vi "S4GUI_001.vi"() -> ()   [LabVIEW 2018] (continued)
                n1814 = call-dynamic "Get CCD_Config.vi"("error in (no error)"=w4172, "Interface in"=w4173) -> ("error out"=w4221:errorcluster, "output cluster"=w4222:T24, "Interface out"=w4218:refnum<class "Interface.lvclass">)  [unwired: 7 in]
                n1815 = Bundle By Name(cluster=w4222, "SHUTTER_MODE"=u8 2, "FRAME_TRANSFER"=w4171) -> (w4220:T24)
                n1816 = call-dynamic "Set CCD_Config.vi"("error in (no error)"=w4221, "input cluster"=w4220, "Interface in"=w4218) -> ("error out"=w4223:errorcluster, "Interface out"=w4217:refnum<class "Interface.lvclass">)  [unwired: 7 in]
                n1817 = Flatten To String(anything=w4220, error in (no error)=w4223) -> (data string=w4225:string, error out=w4224:errorcluster)  [unwired: 2 in, 1 out]
                n1818 = call "Write flatted cluster.vi"("error in (no error)"=w4224, "flatted cluster"=w4225, "Interface in"=w4217) -> ("error out"=w4215:errorcluster, "Interface out"=w4216:refnum<class "Interface.lvclass">)  [unwired: 7 in]
                n1819 = call-dynamic "Write Interface.vi"("error in (no error)"=w4215, "Interface.lvclass"=w4216, "Channel in"=w4229) -> ("error out"=w4210:errorcluster, "Channel out"=w4209:refnum<class "Channel.lvclass">)  [unwired: 7 in]
                n1820 = call "Write section_name.vi"("error in (no error)"=w4210, "section_name"="CCD_ACS4", "Channel in"=w4209) -> ("error out"=w4211:errorcluster, "Channel out"=w4206:refnum<class "Channel.lvclass">)  [unwired: 7 in]
                n1821 = call-dynamic "save config.vi"("error in (no error)"=w4211, "file config"="lastsaved.cfg", "Channel in"=w4206) -> ("error out"=w4179:errorcluster, "Channel out"=w4180:refnum<class "Channel.lvclass">)  [unwired: 7 in]
                n1822 = local read "Filter4"() -> (w4181:u8)
                n1823 = call-dynamic "Write Filter.vi"("error in (no error)"=w4179, "Filter"=w4181, "Channel in"=w4180) -> ("error out"=w4188:errorcluster, "Channel out"=w4189:refnum<class "Channel.lvclass">)  [unwired: 7 in]
                n1824 = call-dynamic "Read Interface.vi"("error in (no error)"=w4188, "Channel in"=w4189) -> ("error out"=w4186:errorcluster, "Interface.lvclass"=w4191:refnum<class "Interface.lvclass">, "Channel out"=w4190:refnum<class "Channel.lvclass">)  [unwired: 7 in]
                n1825 = call-dynamic "Write Suffix.vi"("error in (no error)"=w4186, "Suffix"=w4168, "Interface in"=w4191) -> ("error out"=w4182:errorcluster, "Interface out"=w4192:refnum<class "Interface.lvclass">)  [unwired: 7 in]
                n1826 = call-dynamic "Write ObsType.vi"("error in (no error)"=w4182, "ObsType"=w4167, "Interface in"=w4192) -> ("error out"=w4183:errorcluster, "Interface out"=w4193:refnum<class "Interface.lvclass">)  [unwired: 7 in]
                n1827 = call-dynamic "Write Object.vi"("error in (no error)"=w4183, "Object"=w4176, "Interface in"=w4193) -> ("error out"=w4184:errorcluster, "Interface out"=w4194:refnum<class "Interface.lvclass">)  [unwired: 7 in]
                n1828 = call-dynamic "Write Comments.vi"("error in (no error)"=w4184, "Comments"=w4175, "Interface in"=w4194) -> ("error out"=w4185:errorcluster, "Interface out"=w4195:refnum<class "Interface.lvclass">)  [unwired: 7 in]
                n1829 = call-dynamic "Write Observer.vi"("error in (no error)"=w4185, "Observer"=w4174, "Interface in"=w4195) -> ("error out"=w4187:errorcluster, "Interface out"=w4196:refnum<class "Interface.lvclass">)  [unwired: 7 in]
                n1830 = call-dynamic "Write Interface.vi"("error in (no error)"=w4187, "Interface.lvclass"=w4196, "Channel in"=w4190) -> ("error out"=w4177:errorcluster, "Channel out"=w4178:refnum<class "Channel.lvclass">)  [unwired: 7 in]
                n1831 = call-dynamic "Read State Machine.vi"("error in (no error)"=w4177, "Device in"=w4178) -> ("error out"=w4214:errorcluster, "State Machine.lvclass"=w4204:refnum<class "State Machine.lvclass">, "Device out"=w4205:refnum<class "Channel.lvclass">)  [unwired: 7 in]
                n1832 = call-dynamic "Write State.vi"("error in (no error)"=w4214, "State"=60, "State Machine in"=w4204) -> ("error out"=w4213:errorcluster, "State Machine out"=w4203:refnum<class "State Machine.lvclass">)  [unwired: 7 in]
                n1833 = call-dynamic "Write State Machine.vi"("error in (no error)"=w4213, "State Machine.lvclass"=w4203, "Device in"=w4205) -> ("error out"=w4202:errorcluster, "Device out"=w4197:refnum<class "Channel.lvclass">)  [unwired: 7 in]
                n1834 = call-dynamic "Write Channel.vi"("error in (no error)"=w4202, "Channel.lvclass"=w4197, "Acquisition in"=w4228) -> ("error out"=w4198:errorcluster, "Acquisition out"=w4199:refnum<class "Acquisition.lvclass">)  [unwired: 7 in]
              }
            }
            n1835 = case shown="True" w4144 {
              tunnel: w4146 -> [w4321 w4360]
              tunnel: w4145 -> [w4320 w4359]
              tunnel: [w4321 w4358] -> w4157
              tunnel: [w4320 w4357] -> w4156
              tunnel: w4131 -> [_ w4336]
              tunnel: w4130 -> [_ w4335]
              tunnel: w4129 -> [_ w4334]
              tunnel: w4128 -> [_ w4328]
              tunnel: w4127 -> [_ w4327]
              frame False {
              }
              frame True {
                # "nome do arquivo .cfg"
                # "seção no arquivo .cfg"
                # "closed"
                n1836 = call-dynamic "Read Channel.vi"("error in (no error)"=w4359, "Acquisition in"=w4360) -> ("error out"=w4364:errorcluster, "Channel.lvclass"=w4363:refnum<class "Channel.lvclass">, "Acquisition out"=w4362:refnum<class "Acquisition.lvclass">)  [unwired: 7 in]
                n1837 = call-dynamic "Read Interface.vi"("error in (no error)"=w4364, "Channel in"=w4363) -> ("error out"=w4326:errorcluster, "Interface.lvclass"=w4325:refnum<class "Interface.lvclass">, "Channel out"=w4361:refnum<class "Channel.lvclass">)  [unwired: 7 in]
                n1838 = call-dynamic "Read restoreExpTime.vi"("error in (no error)"=w4326, "Interface in"=w4325) -> ("error out"=w4323:errorcluster, "restoreExpTime"=w4322:bool, "Interface out"=w4324:refnum<class "Interface.lvclass">)  [unwired: 7 in]
                n1839 = case shown="True" w4322 {
                  tunnel: w4324 -> [w4391 w4396]
                  tunnel: [w4391 w4399] -> w4330
                  tunnel: w4323 -> [w4390 w4394]
                  tunnel: [w4390 w4398] -> w4329
                  frame False {
                  }
                  frame True {
                    n1840 = call-dynamic "Write restoreExpTime.vi"("error in (no error)"=w4394, "restoreExpTime"=FALSE, "Interface in"=w4396) -> ("error out"=w4393:errorcluster, "Interface out"=w4395:refnum<class "Interface.lvclass">)  [unwired: 7 in]
                    n1841 = call-dynamic "Read prev ExpTime.vi"("error in (no error)"=w4393, "Interface in"=w4395) -> ("error out"=w4398:errorcluster, "prev ExpTime"=w4397:dbl, "Interface out"=w4399:refnum<class "Interface.lvclass">)  [unwired: 7 in]
                    n1842 = property on="Exptime ch2" class="DigNum (strict)"("Value"=w4397) -> ()  [unwired: 2 in, 2 out]
                  }
                }
                n1843 = call-dynamic "Read PREV_FT.vi"("error in (no error)"=w4329, "Interface in"=w4330) -> ("error out"=w4332:errorcluster, "PREV_FT"=w4331:bool, "Interface out"=w4333:refnum<class "Interface.lvclass">)  [unwired: 7 in]
                n1844 = call-dynamic "Get CCD_Config.vi"("error in (no error)"=w4332, "Interface in"=w4333) -> ("error out"=w4369:errorcluster, "output cluster"=w4368:T24, "Interface out"=w4372:refnum<class "Interface.lvclass">)  [unwired: 7 in]
                n1845 = Bundle By Name(cluster=w4368, "SHUTTER_MODE"=u8 2, "FRAME_TRANSFER"=w4331) -> (w4370:T24)
                n1846 = call-dynamic "Set CCD_Config.vi"("error in (no error)"=w4369, "input cluster"=w4370, "Interface in"=w4372) -> ("error out"=w4367:errorcluster, "Interface out"=w4373:refnum<class "Interface.lvclass">)  [unwired: 7 in]
                n1847 = Flatten To String(anything=w4370, error in (no error)=w4367) -> (data string=w4365:string, error out=w4366:errorcluster)  [unwired: 2 in, 1 out]
                n1848 = call "Write flatted cluster.vi"("error in (no error)"=w4366, "flatted cluster"=w4365, "Interface in"=w4373) -> ("error out"=w4375:errorcluster, "Interface out"=w4374:refnum<class "Interface.lvclass">)  [unwired: 7 in]
                n1849 = call-dynamic "Write Interface.vi"("error in (no error)"=w4375, "Interface.lvclass"=w4374, "Channel in"=w4361) -> ("error out"=w4380:errorcluster, "Channel out"=w4381:refnum<class "Channel.lvclass">)  [unwired: 7 in]
                n1850 = call "Write section_name.vi"("error in (no error)"=w4380, "section_name"="CCD_ACS2", "Channel in"=w4381) -> ("error out"=w4379:errorcluster, "Channel out"=w4384:refnum<class "Channel.lvclass">)  [unwired: 7 in]
                n1851 = call-dynamic "save config.vi"("error in (no error)"=w4379, "file config"="lastsaved.cfg", "Channel in"=w4384) -> ("error out"=w4339:errorcluster, "Channel out"=w4340:refnum<class "Channel.lvclass">)  [unwired: 7 in]
                n1852 = local read "Filter2"() -> (w4341:u8)
                n1853 = call-dynamic "Write Filter.vi"("error in (no error)"=w4339, "Filter"=w4341, "Channel in"=w4340) -> ("error out"=w4348:errorcluster, "Channel out"=w4349:refnum<class "Channel.lvclass">)  [unwired: 7 in]
                n1854 = call-dynamic "Read Interface.vi"("error in (no error)"=w4348, "Channel in"=w4349) -> ("error out"=w4346:errorcluster, "Interface.lvclass"=w4351:refnum<class "Interface.lvclass">, "Channel out"=w4350:refnum<class "Channel.lvclass">)  [unwired: 7 in]
                n1855 = call-dynamic "Write Suffix.vi"("error in (no error)"=w4346, "Suffix"=w4328, "Interface in"=w4351) -> ("error out"=w4342:errorcluster, "Interface out"=w4352:refnum<class "Interface.lvclass">)  [unwired: 7 in]
                n1856 = call-dynamic "Write ObsType.vi"("error in (no error)"=w4342, "ObsType"=w4327, "Interface in"=w4352) -> ("error out"=w4343:errorcluster, "Interface out"=w4353:refnum<class "Interface.lvclass">)  [unwired: 7 in]
                n1857 = call-dynamic "Write Object.vi"("error in (no error)"=w4343, "Object"=w4336, "Interface in"=w4353) -> ("error out"=w4344:errorcluster, "Interface out"=w4354:refnum<class "Interface.lvclass">)  [unwired: 7 in]
                n1858 = call-dynamic "Write Comments.vi"("error in (no error)"=w4344, "Comments"=w4335, "Interface in"=w4354) -> ("error out"=w4345:errorcluster, "Interface out"=w4355:refnum<class "Interface.lvclass">)  [unwired: 7 in]
                n1859 = call-dynamic "Write Observer.vi"("error in (no error)"=w4345, "Observer"=w4334, "Interface in"=w4355) -> ("error out"=w4347:errorcluster, "Interface out"=w4356:refnum<class "Interface.lvclass">)  [unwired: 7 in]
                n1860 = call-dynamic "Write Interface.vi"("error in (no error)"=w4347, "Interface.lvclass"=w4356, "Channel in"=w4350) -> ("error out"=w4337:errorcluster, "Channel out"=w4338:refnum<class "Channel.lvclass">)  [unwired: 7 in]
                n1861 = call-dynamic "Read State Machine.vi"("error in (no error)"=w4337, "Device in"=w4338) -> ("error out"=w4376:errorcluster, "State Machine.lvclass"=w4386:refnum<class "State Machine.lvclass">, "Device out"=w4385:refnum<class "Channel.lvclass">)  [unwired: 7 in]
                n1862 = call-dynamic "Write State.vi"("error in (no error)"=w4376, "State"=60, "State Machine in"=w4386) -> ("error out"=w4377:errorcluster, "State Machine out"=w4387:refnum<class "State Machine.lvclass">)  [unwired: 7 in]
                n1863 = call-dynamic "Write State Machine.vi"("error in (no error)"=w4377, "State Machine.lvclass"=w4387, "Device in"=w4385) -> ("error out"=w4389:errorcluster, "Device out"=w4388:refnum<class "Channel.lvclass">)  [unwired: 7 in]
                n1864 = call-dynamic "Write Channel.vi"("error in (no error)"=w4389, "Channel.lvclass"=w4388, "Acquisition in"=w4362) -> ("error out"=w4357:errorcluster, "Acquisition out"=w4358:refnum<class "Acquisition.lvclass">)  [unwired: 7 in]
              }
            }
            n1865 = case shown="True" w4141 {
              tunnel: w4143 -> [w4241 w4280]
              tunnel: w4142 -> [w4240 w4279]
              tunnel: [w4241 w4278] -> w4155
              tunnel: [w4240 w4277] -> w4154
              tunnel: w4131 -> [_ w4256]
              tunnel: w4130 -> [_ w4255]
              tunnel: w4129 -> [_ w4254]
              tunnel: w4128 -> [_ w4248]
              tunnel: w4127 -> [_ w4247]
              frame False {
              }
              frame True {
                # "nome do arquivo .cfg"
                # "seção no arquivo .cfg"
                # "closed"
                n1866 = call-dynamic "Read Channel.vi"("error in (no error)"=w4279, "Acquisition in"=w4280) -> ("error out"=w4284:errorcluster, "Channel.lvclass"=w4283:refnum<class "Channel.lvclass">, "Acquisition out"=w4282:refnum<class "Acquisition.lvclass">)  [unwired: 7 in]
                n1867 = call-dynamic "Read Interface.vi"("error in (no error)"=w4284, "Channel in"=w4283) -> ("error out"=w4244:errorcluster, "Interface.lvclass"=w4246:refnum<class "Interface.lvclass">, "Channel out"=w4281:refnum<class "Channel.lvclass">)  [unwired: 7 in]
                n1868 = call-dynamic "Read restoreExpTime.vi"("error in (no error)"=w4244, "Interface in"=w4246) -> ("error out"=w4243:errorcluster, "restoreExpTime"=w4242:bool, "Interface out"=w4245:refnum<class "Interface.lvclass">)  [unwired: 7 in]
                n1869 = case shown="True" w4242 {
                  tunnel: w4245 -> [w4311 w4316]
                  tunnel: [w4311 w4319] -> w4250
                  tunnel: w4243 -> [w4310 w4315]
                  tunnel: [w4310 w4318] -> w4249
                  frame False {
                  }
                  frame True {
                    n1870 = call-dynamic "Write restoreExpTime.vi"("error in (no error)"=w4315, "restoreExpTime"=FALSE, "Interface in"=w4316) -> ("error out"=w4312:errorcluster, "Interface out"=w4313:refnum<class "Interface.lvclass">)  [unwired: 7 in]
                    n1871 = call-dynamic "Read prev ExpTime.vi"("error in (no error)"=w4312, "Interface in"=w4313) -> ("error out"=w4318:errorcluster, "prev ExpTime"=w4317:dbl, "Interface out"=w4319:refnum<class "Interface.lvclass">)  [unwired: 7 in]
                    n1872 = property on="Exptime ch3" class="DigNum (strict)"("Value"=w4317) -> ()  [unwired: 2 in, 2 out]
                  }
                }
                n1873 = call-dynamic "Read PREV_FT.vi"("error in (no error)"=w4249, "Interface in"=w4250) -> ("error out"=w4252:errorcluster, "PREV_FT"=w4251:bool, "Interface out"=w4253:refnum<class "Interface.lvclass">)  [unwired: 7 in]
                n1874 = call-dynamic "Get CCD_Config.vi"("error in (no error)"=w4252, "Interface in"=w4253) -> ("error out"=w4289:errorcluster, "output cluster"=w4288:T24, "Interface out"=w4292:refnum<class "Interface.lvclass">)  [unwired: 7 in]
                n1875 = Bundle By Name(cluster=w4288, "SHUTTER_MODE"=u8 2, "FRAME_TRANSFER"=w4251) -> (w4290:T24)
                n1876 = call-dynamic "Set CCD_Config.vi"("error in (no error)"=w4289, "input cluster"=w4290, "Interface in"=w4292) -> ("error out"=w4287:errorcluster, "Interface out"=w4293:refnum<class "Interface.lvclass">)  [unwired: 7 in]
                n1877 = Flatten To String(anything=w4290, error in (no error)=w4287) -> (data string=w4285:string, error out=w4286:errorcluster)  [unwired: 2 in, 1 out]
                n1878 = call "Write flatted cluster.vi"("error in (no error)"=w4286, "flatted cluster"=w4285, "Interface in"=w4293) -> ("error out"=w4295:errorcluster, "Interface out"=w4294:refnum<class "Interface.lvclass">)  [unwired: 7 in]
                n1879 = call-dynamic "Write Interface.vi"("error in (no error)"=w4295, "Interface.lvclass"=w4294, "Channel in"=w4281) -> ("error out"=w4300:errorcluster, "Channel out"=w4301:refnum<class "Channel.lvclass">)  [unwired: 7 in]
                n1880 = call "Write section_name.vi"("error in (no error)"=w4300, "section_name"="CCD_ACS3", "Channel in"=w4301) -> ("error out"=w4299:errorcluster, "Channel out"=w4304:refnum<class "Channel.lvclass">)  [unwired: 7 in]
                n1881 = call-dynamic "save config.vi"("error in (no error)"=w4299, "file config"="lastsaved.cfg", "Channel in"=w4304) -> ("error out"=w4259:errorcluster, "Channel out"=w4260:refnum<class "Channel.lvclass">)  [unwired: 7 in]
                n1882 = local read "Filter3"() -> (w4261:u8)
                n1883 = call-dynamic "Write Filter.vi"("error in (no error)"=w4259, "Filter"=w4261, "Channel in"=w4260) -> ("error out"=w4268:errorcluster, "Channel out"=w4269:refnum<class "Channel.lvclass">)  [unwired: 7 in]
                n1884 = call-dynamic "Read Interface.vi"("error in (no error)"=w4268, "Channel in"=w4269) -> ("error out"=w4266:errorcluster, "Interface.lvclass"=w4271:refnum<class "Interface.lvclass">, "Channel out"=w4270:refnum<class "Channel.lvclass">)  [unwired: 7 in]
                n1885 = call-dynamic "Write Suffix.vi"("error in (no error)"=w4266, "Suffix"=w4248, "Interface in"=w4271) -> ("error out"=w4262:errorcluster, "Interface out"=w4272:refnum<class "Interface.lvclass">)  [unwired: 7 in]
                n1886 = call-dynamic "Write ObsType.vi"("error in (no error)"=w4262, "ObsType"=w4247, "Interface in"=w4272) -> ("error out"=w4263:errorcluster, "Interface out"=w4273:refnum<class "Interface.lvclass">)  [unwired: 7 in]
                n1887 = call-dynamic "Write Object.vi"("error in (no error)"=w4263, "Object"=w4256, "Interface in"=w4273) -> ("error out"=w4264:errorcluster, "Interface out"=w4274:refnum<class "Interface.lvclass">)  [unwired: 7 in]
                n1888 = call-dynamic "Write Comments.vi"("error in (no error)"=w4264, "Comments"=w4255, "Interface in"=w4274) -> ("error out"=w4265:errorcluster, "Interface out"=w4275:refnum<class "Interface.lvclass">)  [unwired: 7 in]
                n1889 = call-dynamic "Write Observer.vi"("error in (no error)"=w4265, "Observer"=w4254, "Interface in"=w4275) -> ("error out"=w4267:errorcluster, "Interface out"=w4276:refnum<class "Interface.lvclass">)  [unwired: 7 in]
                n1890 = call-dynamic "Write Interface.vi"("error in (no error)"=w4267, "Interface.lvclass"=w4276, "Channel in"=w4270) -> ("error out"=w4257:errorcluster, "Channel out"=w4258:refnum<class "Channel.lvclass">)  [unwired: 7 in]
                n1891 = call-dynamic "Read State Machine.vi"("error in (no error)"=w4257, "Device in"=w4258) -> ("error out"=w4296:errorcluster, "State Machine.lvclass"=w4306:refnum<class "State Machine.lvclass">, "Device out"=w4305:refnum<class "Channel.lvclass">)  [unwired: 7 in]
                n1892 = call-dynamic "Write State.vi"("error in (no error)"=w4296, "State"=60, "State Machine in"=w4306) -> ("error out"=w4297:errorcluster, "State Machine out"=w4307:refnum<class "State Machine.lvclass">)  [unwired: 7 in]
                n1893 = call-dynamic "Write State Machine.vi"("error in (no error)"=w4297, "State Machine.lvclass"=w4307, "Device in"=w4305) -> ("error out"=w4309:errorcluster, "Device out"=w4308:refnum<class "Channel.lvclass">)  [unwired: 7 in]
                n1894 = call-dynamic "Write Channel.vi"("error in (no error)"=w4309, "Channel.lvclass"=w4308, "Acquisition in"=w4282) -> ("error out"=w4277:errorcluster, "Acquisition out"=w4278:refnum<class "Acquisition.lvclass">)  [unwired: 7 in]
              }
            }
            n1895 = case shown="True" w4147 {
              tunnel: [w4400 w4465] -> w4158
              tunnel: [w4401 w4464] -> w4159
              tunnel: w4149 -> [w4401 w4438]
              tunnel: w4148 -> [w4400 w4437]
              tunnel: w4131 -> [_ w4416]
              tunnel: w4130 -> [_ w4415]
              tunnel: w4129 -> [_ w4414]
              tunnel: w4128 -> [_ w4408]
              tunnel: w4127 -> [_ w4407]
              frame False {
              }
              frame True {
                # "nome do arquivo .cfg"
                # "seção no arquivo .cfg"
                # "closed"
                n1896 = call-dynamic "Read Channel.vi"("error in (no error)"=w4437, "Acquisition in"=w4438) -> ("error out"=w4466:errorcluster, "Channel.lvclass"=w4467:refnum<class "Channel.lvclass">, "Acquisition out"=w4468:refnum<class "Acquisition.lvclass">)  [unwired: 7 in]
                n1897 = call-dynamic "Read Interface.vi"("error in (no error)"=w4466, "Channel in"=w4467) -> ("error out"=w4405:errorcluster, "Interface.lvclass"=w4406:refnum<class "Interface.lvclass">, "Channel out"=w4469:refnum<class "Channel.lvclass">)  [unwired: 7 in]
                n1898 = call-dynamic "Read restoreExpTime.vi"("error in (no error)"=w4405, "Interface in"=w4406) -> ("error out"=w4403:errorcluster, "restoreExpTime"=w4402:bool, "Interface out"=w4404:refnum<class "Interface.lvclass">)  [unwired: 7 in]
                n1899 = case shown="True" w4402 {
                  tunnel: [w4471 w4479] -> w4410
                  tunnel: [w4470 w4478] -> w4409
                  tunnel: w4404 -> [w4471 w4476]
                  tunnel: w4403 -> [w4470 w4474]
                  frame False {
                  }
                  frame True {
                    n1900 = call-dynamic "Write restoreExpTime.vi"("error in (no error)"=w4474, "restoreExpTime"=FALSE, "Interface in"=w4476) -> ("error out"=w4473:errorcluster, "Interface out"=w4475:refnum<class "Interface.lvclass">)  [unwired: 7 in]
                    n1901 = call-dynamic "Read prev ExpTime.vi"("error in (no error)"=w4473, "Interface in"=w4475) -> ("error out"=w4478:errorcluster, "prev ExpTime"=w4477:dbl, "Interface out"=w4479:refnum<class "Interface.lvclass">)  [unwired: 7 in]
                    n1902 = property on="Exptime ch1" class="DigNum (strict)"("Value"=w4477) -> ()  [unwired: 2 in, 2 out]
                  }
                }
                n1903 = call-dynamic "Read PREV_FT.vi"("error in (no error)"=w4409, "Interface in"=w4410) -> ("error out"=w4412:errorcluster, "PREV_FT"=w4411:bool, "Interface out"=w4413:refnum<class "Interface.lvclass">)  [unwired: 7 in]
                n1904 = call-dynamic "Get CCD_Config.vi"("error in (no error)"=w4412, "Interface in"=w4413) -> ("error out"=w4459:errorcluster, "output cluster"=w4460:T24, "Interface out"=w4456:refnum<class "Interface.lvclass">)  [unwired: 7 in]
                n1905 = Bundle By Name(cluster=w4460, "SHUTTER_MODE"=u8 2, "FRAME_TRANSFER"=w4411) -> (w4458:T24)
                n1906 = call-dynamic "Set CCD_Config.vi"("error in (no error)"=w4459, "input cluster"=w4458, "Interface in"=w4456) -> ("error out"=w4461:errorcluster, "Interface out"=w4455:refnum<class "Interface.lvclass">)  [unwired: 7 in]
                n1907 = Flatten To String(anything=w4458, error in (no error)=w4461) -> (data string=w4463:string, error out=w4462:errorcluster)  [unwired: 2 in, 1 out]
                n1908 = call "Write flatted cluster.vi"("error in (no error)"=w4462, "flatted cluster"=w4463, "Interface in"=w4455) -> ("error out"=w4453:errorcluster, "Interface out"=w4454:refnum<class "Interface.lvclass">)  [unwired: 7 in]
                n1909 = call-dynamic "Write Interface.vi"("error in (no error)"=w4453, "Interface.lvclass"=w4454, "Channel in"=w4469) -> ("error out"=w4448:errorcluster, "Channel out"=w4447:refnum<class "Channel.lvclass">)  [unwired: 7 in]
                n1910 = call "Write section_name.vi"("error in (no error)"=w4448, "section_name"="CCD_ACS1", "Channel in"=w4447) -> ("error out"=w4449:errorcluster, "Channel out"=w4444:refnum<class "Channel.lvclass">)  [unwired: 7 in]
                n1911 = call-dynamic "save config.vi"("error in (no error)"=w4449, "file config"="lastsaved.cfg", "Channel in"=w4444) -> ("error out"=w4419:errorcluster, "Channel out"=w4420:refnum<class "Channel.lvclass">)  [unwired: 7 in]
                n1912 = local read "Filter1"() -> (w4421:u8)
                n1913 = call-dynamic "Write Filter.vi"("error in (no error)"=w4419, "Filter"=w4421, "Channel in"=w4420) -> ("error out"=w4428:errorcluster, "Channel out"=w4429:refnum<class "Channel.lvclass">)  [unwired: 7 in]
                n1914 = call-dynamic "Read Interface.vi"("error in (no error)"=w4428, "Channel in"=w4429) -> ("error out"=w4426:errorcluster, "Interface.lvclass"=w4431:refnum<class "Interface.lvclass">, "Channel out"=w4430:refnum<class "Channel.lvclass">)  [unwired: 7 in]
                n1915 = call-dynamic "Write Suffix.vi"("error in (no error)"=w4426, "Suffix"=w4408, "Interface in"=w4431) -> ("error out"=w4422:errorcluster, "Interface out"=w4432:refnum<class "Interface.lvclass">)  [unwired: 7 in]
                n1916 = call-dynamic "Write ObsType.vi"("error in (no error)"=w4422, "ObsType"=w4407, "Interface in"=w4432) -> ("error out"=w4423:errorcluster, "Interface out"=w4433:refnum<class "Interface.lvclass">)  [unwired: 7 in]
                n1917 = call-dynamic "Write Object.vi"("error in (no error)"=w4423, "Object"=w4416, "Interface in"=w4433) -> ("error out"=w4424:errorcluster, "Interface out"=w4434:refnum<class "Interface.lvclass">)  [unwired: 7 in]
                n1918 = call-dynamic "Write Comments.vi"("error in (no error)"=w4424, "Comments"=w4415, "Interface in"=w4434) -> ("error out"=w4425:errorcluster, "Interface out"=w4435:refnum<class "Interface.lvclass">)  [unwired: 7 in]
                n1919 = call-dynamic "Write Observer.vi"("error in (no error)"=w4425, "Observer"=w4414, "Interface in"=w4435) -> ("error out"=w4427:errorcluster, "Interface out"=w4436:refnum<class "Interface.lvclass">)  [unwired: 7 in]
                n1920 = call-dynamic "Write Interface.vi"("error in (no error)"=w4427, "Interface.lvclass"=w4436, "Channel in"=w4430) -> ("error out"=w4417:errorcluster, "Channel out"=w4418:refnum<class "Channel.lvclass">)  [unwired: 7 in]
                n1921 = call-dynamic "Read State Machine.vi"("error in (no error)"=w4417, "Device in"=w4418) -> ("error out"=w4452:errorcluster, "State Machine.lvclass"=w4442:refnum<class "State Machine.lvclass">, "Device out"=w4443:refnum<class "Channel.lvclass">)  [unwired: 7 in]
                n1922 = call-dynamic "Write State.vi"("error in (no error)"=w4452, "State"=60, "State Machine in"=w4442) -> ("error out"=w4451:errorcluster, "State Machine out"=w4441:refnum<class "State Machine.lvclass">)  [unwired: 7 in]
                n1923 = call-dynamic "Write State Machine.vi"("error in (no error)"=w4451, "State Machine.lvclass"=w4441, "Device in"=w4443) -> ("error out"=w4439:errorcluster, "Device out"=w4440:refnum<class "Channel.lvclass">)  [unwired: 7 in]
                n1924 = call-dynamic "Write Channel.vi"("error in (no error)"=w4439, "Channel.lvclass"=w4440, "Acquisition in"=w4468) -> ("error out"=w4465:errorcluster, "Acquisition out"=w4464:refnum<class "Acquisition.lvclass">)  [unwired: 7 in]
              }
            }
          }
          frame "OBJECT", Default {
            # "OBJECT, DFLAT,SFLAT and FOCUS: Shutter automatically open and restore FRAME_TRANSFER."
            n1925 = call "Read connection.vi"("error in (no error)"=w4503, "Server in"=w4504) -> ("error out"=w4501:errorcluster, "connection"=w4500:bool, "Server out"=w4502:refnum<class "Acquisition.lvclass">)  [unwired: 7 in]
            n1926 = call "Read connection.vi"("error in (no error)"=w4485, "Server in"=w4486) -> ("error out"=w4492:errorcluster, "connection"=w4491:bool, "Server out"=w4493:refnum<class "Acquisition.lvclass">)  [unwired: 7 in]
            n1927 = call "Read connection.vi"("error in (no error)"=w4487, "Server in"=w4488) -> ("error out"=w4495:errorcluster, "connection"=w4494:bool, "Server out"=w4496:refnum<class "Acquisition.lvclass">)  [unwired: 7 in]
            n1928 = call "Read connection.vi"("error in (no error)"=w4489, "Server in"=w4490) -> ("error out"=w4498:errorcluster, "connection"=w4497:bool, "Server out"=w4499:refnum<class "Acquisition.lvclass">)  [unwired: 7 in]
            n1929 = case shown="True" w4491 {
              tunnel: w4493 -> [w4514 w4553]
              tunnel: w4492 -> [w4513 w4552]
              tunnel: [w4514 w4551] -> w4506
              tunnel: [w4513 w4550] -> w4505
              tunnel: w4484 -> [_ w4530]
              tunnel: w4483 -> [_ w4529]
              tunnel: w4482 -> [_ w4528]
              tunnel: w4481 -> [_ w4521]
              tunnel: w4480 -> [_ w4520]
              frame False {
              }
              frame True {
                # "nome do arquivo .cfg"
                # "seção no arquivo .cfg"
                # "open"
                n1930 = call-dynamic "Read Channel.vi"("error in (no error)"=w4552, "Acquisition in"=w4553) -> ("error out"=w4578:errorcluster, "Channel.lvclass"=w4579:refnum<class "Channel.lvclass">, "Acquisition out"=w4580:refnum<class "Acquisition.lvclass">)  [unwired: 7 in]
                n1931 = call-dynamic "Read Interface.vi"("error in (no error)"=w4578, "Channel in"=w4579) -> ("error out"=w4517:errorcluster, "Interface.lvclass"=w4518:refnum<class "Interface.lvclass">, "Channel out"=w4581:refnum<class "Channel.lvclass">)  [unwired: 7 in]
                n1932 = call-dynamic "Read restoreExpTime.vi"("error in (no error)"=w4517, "Interface in"=w4518) -> ("error out"=w4516:errorcluster, "restoreExpTime"=w4519:bool, "Interface out"=w4515:refnum<class "Interface.lvclass">)  [unwired: 7 in]
                n1933 = case shown="True" w4519 {
                  tunnel: w4515 -> [w4583 w4588]
                  tunnel: [w4583 w4591] -> w4524
                  tunnel: w4516 -> [w4582 w4587]
                  tunnel: [w4582 w4590] -> w4523
                  frame False {
                  }
                  frame True {
                    n1934 = call-dynamic "Write restoreExpTime.vi"("error in (no error)"=w4587, "restoreExpTime"=FALSE, "Interface in"=w4588) -> ("error out"=w4585:errorcluster, "Interface out"=w4586:refnum<class "Interface.lvclass">)  [unwired: 7 in]
                    n1935 = call-dynamic "Read prev ExpTime.vi"("error in (no error)"=w4585, "Interface in"=w4586) -> ("error out"=w4590:errorcluster, "prev ExpTime"=w4589:dbl, "Interface out"=w4591:refnum<class "Interface.lvclass">)  [unwired: 7 in]
                    n1936 = property on="Exptime ch4" class="DigNum (strict)"("Value"=w4589) -> ()  [unwired: 2 in, 2 out]
                  }
                }
                n1937 = call-dynamic "Read PREV_FT.vi"("error in (no error)"=w4523, "Interface in"=w4524) -> ("error out"=w4526:errorcluster, "PREV_FT"=w4525:bool, "Interface out"=w4527:refnum<class "Interface.lvclass">)  [unwired: 7 in]
                n1938 = call-dynamic "Get CCD_Config.vi"("error in (no error)"=w4526, "Interface in"=w4527) -> ("error out"=w4573:errorcluster, "output cluster"=w4574:T24, "Interface out"=w4570:refnum<class "Interface.lvclass">)  [unwired: 7 in]
                n1939 = Bundle By Name(cluster=w4574, "SHUTTER_MODE"=u8 1, "FRAME_TRANSFER"=w4525) -> (w4572:T24)
                n1940 = call-dynamic "Set CCD_Config.vi"("error in (no error)"=w4573, "input cluster"=w4572, "Interface in"=w4570) -> ("error out"=w4575:errorcluster, "Interface out"=w4569:refnum<class "Interface.lvclass">)  [unwired: 7 in]
                n1941 = Flatten To String(anything=w4572, error in (no error)=w4575) -> (data string=w4577:string, error out=w4576:errorcluster)  [unwired: 2 in, 1 out]
                n1942 = call "Write flatted cluster.vi"("error in (no error)"=w4576, "flatted cluster"=w4577, "Interface in"=w4569) -> ("error out"=w4567:errorcluster, "Interface out"=w4568:refnum<class "Interface.lvclass">)  [unwired: 7 in]
                n1943 = call-dynamic "Write Interface.vi"("error in (no error)"=w4567, "Interface.lvclass"=w4568, "Channel in"=w4581) -> ("error out"=w4563:errorcluster, "Channel out"=w4562:refnum<class "Channel.lvclass">)  [unwired: 7 in]
                n1944 = call "Write section_name.vi"("error in (no error)"=w4563, "section_name"="CCD_ACS4", "Channel in"=w4562) -> ("error out"=w4564:errorcluster, "Channel out"=w4559:refnum<class "Channel.lvclass">)  [unwired: 7 in]
                n1945 = call-dynamic "save config.vi"("error in (no error)"=w4564, "file config"="lastsaved.cfg", "Channel in"=w4559) -> ("error out"=w4532:errorcluster, "Channel out"=w4536:refnum<class "Channel.lvclass">)  [unwired: 7 in]
                n1946 = local read "Filter4"() -> (w4531:u8)
                n1947 = call-dynamic "Write Filter.vi"("error in (no error)"=w4532, "Filter"=w4531, "Channel in"=w4536) -> ("error out"=w4549:errorcluster, "Channel out"=w4535:refnum<class "Channel.lvclass">)  [unwired: 7 in]
                n1948 = call-dynamic "Read Interface.vi"("error in (no error)"=w4549, "Channel in"=w4535) -> ("error out"=w4546:errorcluster, "Interface.lvclass"=w4545:refnum<class "Interface.lvclass">, "Channel out"=w4534:refnum<class "Channel.lvclass">)  [unwired: 7 in]
                n1949 = call-dynamic "Write Suffix.vi"("error in (no error)"=w4546, "Suffix"=w4521, "Interface in"=w4545) -> ("error out"=w4537:errorcluster, "Interface out"=w4540:refnum<class "Interface.lvclass">)  [unwired: 7 in]
                n1950 = call-dynamic "Write ObsType.vi"("error in (no error)"=w4537, "ObsType"=w4520, "Interface in"=w4540) -> ("error out"=w4538:errorcluster, "Interface out"=w4541:refnum<class "Interface.lvclass">)  [unwired: 7 in]
                n1951 = call-dynamic "Write Object.vi"("error in (no error)"=w4538, "Object"=w4530, "Interface in"=w4541) -> ("error out"=w4539:errorcluster, "Interface out"=w4542:refnum<class "Interface.lvclass">)  [unwired: 7 in]
                n1952 = call-dynamic "Write Comments.vi"("error in (no error)"=w4539, "Comments"=w4529, "Interface in"=w4542) -> ("error out"=w4543:errorcluster, "Interface out"=w4544:refnum<class "Interface.lvclass">)  [unwired: 7 in]
                n1953 = call-dynamic "Write Observer.vi"("error in (no error)"=w4543, "Observer"=w4528, "Interface in"=w4544) -> ("error out"=w4548:errorcluster, "Interface out"=w4547:refnum<class "Interface.lvclass">)  [unwired: 7 in]
                n1954 = call-dynamic "Write Interface.vi"("error in (no error)"=w4548, "Interface.lvclass"=w4547, "Channel in"=w4534) -> ("error out"=w4522:errorcluster, "Channel out"=w4533:refnum<class "Channel.lvclass">)  [unwired: 7 in]
                n1955 = call-dynamic "Read State Machine.vi"("error in (no error)"=w4522, "Device in"=w4533) -> ("State Machine.lvclass"=w4557:refnum<class "State Machine.lvclass">, "Device out"=w4558:refnum<class "Channel.lvclass">)  [unwired: 7 in, 1 out]
                n1956 = call-dynamic "Write State.vi"("error in (no error)"=w4522, "State"=60, "State Machine in"=w4557) -> ("error out"=w4566:errorcluster, "State Machine out"=w4556:refnum<class "State Machine.lvclass">)  [unwired: 7 in]
                n1957 = call-dynamic "Write State Machine.vi"("error in (no error)"=w4566, "State Machine.lvclass"=w4556, "Device in"=w4558) -> ("error out"=w4554:errorcluster, "Device out"=w4555:refnum<class "Channel.lvclass">)  [unwired: 7 in]
                n1958 = call-dynamic "Write Channel.vi"("error in (no error)"=w4554, "Channel.lvclass"=w4555, "Acquisition in"=w4580) -> ("error out"=w4550:errorcluster, "Acquisition out"=w4551:refnum<class "Acquisition.lvclass">)  [unwired: 7 in]
              }
            }
            n1959 = case shown="True" w4500 {
              tunnel: [w4752 w4817] -> w4511
              tunnel: [w4753 w4816] -> w4512
              tunnel: w4502 -> [w4753 w4790]
              tunnel: w4501 -> [w4752 w4789]
              tunnel: w4484 -> [_ w4768]
              tunnel: w4483 -> [_ w4767]
              tunnel: w4482 -> [_ w4766]
              tunnel: w4481 -> [_ w4760]
              tunnel: w4480 -> [_ w4759]
              frame False {
              }
              frame True {
                # "nome do arquivo .cfg"
                # "seção no arquivo .cfg"
                # "open"
                n1960 = call-dynamic "Read Channel.vi"("error in (no error)"=w4789, "Acquisition in"=w4790) -> ("error out"=w4818:errorcluster, "Channel.lvclass"=w4819:refnum<class "Channel.lvclass">, "Acquisition out"=w4820:refnum<class "Acquisition.lvclass">)  [unwired: 7 in]
                n1961 = call-dynamic "Read Interface.vi"("error in (no error)"=w4818, "Channel in"=w4819) -> ("error out"=w4757:errorcluster, "Interface.lvclass"=w4758:refnum<class "Interface.lvclass">, "Channel out"=w4821:refnum<class "Channel.lvclass">)  [unwired: 7 in]
                n1962 = call-dynamic "Read restoreExpTime.vi"("error in (no error)"=w4757, "Interface in"=w4758) -> ("error out"=w4755:errorcluster, "restoreExpTime"=w4754:bool, "Interface out"=w4756:refnum<class "Interface.lvclass">)  [unwired: 7 in]
                n1963 = case shown="True" w4754 {
                  tunnel: w4756 -> [w4823 w4828]
                  tunnel: [w4823 w4831] -> w4762
                  tunnel: w4755 -> [w4822 w4826]
                  tunnel: [w4822 w4830] -> w4761
                  frame False {
                  }
                  frame True {
                    n1964 = call-dynamic "Write restoreExpTime.vi"("error in (no error)"=w4826, "restoreExpTime"=FALSE, "Interface in"=w4828) -> ("error out"=w4825:errorcluster, "Interface out"=w4827:refnum<class "Interface.lvclass">)  [unwired: 7 in]
                    n1965 = call-dynamic "Read prev ExpTime.vi"("error in (no error)"=w4825, "Interface in"=w4827) -> ("error out"=w4830:errorcluster, "prev ExpTime"=w4829:dbl, "Interface out"=w4831:refnum<class "Interface.lvclass">)  [unwired: 7 in]
                    n1966 = property on="Exptime ch1" class="DigNum (strict)"("Value"=w4829) -> ()  [unwired: 2 in, 2 out]
                  }
                }
                n1967 = call-dynamic "Read PREV_FT.vi"("error in (no error)"=w4761, "Interface in"=w4762) -> ("error out"=w4764:errorcluster, "PREV_FT"=w4763:bool, "Interface out"=w4765:refnum<class "Interface.lvclass">)  [unwired: 7 in]
                n1968 = call-dynamic "Get CCD_Config.vi"("error in (no error)"=w4764, "Interface in"=w4765) -> ("error out"=w4811:errorcluster, "output cluster"=w4812:T24, "Interface out"=w4808:refnum<class "Interface.lvclass">)  [unwired: 7 in]
                n1969 = Bundle By Name(cluster=w4812, "SHUTTER_MODE"=u8 1, "FRAME_TRANSFER"=w4763) -> (w4810:T24)
                n1970 = call-dynamic "Set CCD_Config.vi"("error in (no error)"=w4811, "input cluster"=w4810, "Interface in"=w4808) -> ("error out"=w4813:errorcluster, "Interface out"=w4807:refnum<class "Interface.lvclass">)  [unwired: 7 in]
                n1971 = Flatten To String(anything=w4810, error in (no error)=w4813) -> (data string=w4815:string, error out=w4814:errorcluster)  [unwired: 2 in, 1 out]
                n1972 = call "Write flatted cluster.vi"("error in (no error)"=w4814, "flatted cluster"=w4815, "Interface in"=w4807) -> ("error out"=w4805:errorcluster, "Interface out"=w4806:refnum<class "Interface.lvclass">)  [unwired: 7 in]
                n1973 = call-dynamic "Write Interface.vi"("error in (no error)"=w4805, "Interface.lvclass"=w4806, "Channel in"=w4821) -> ("error out"=w4800:errorcluster, "Channel out"=w4799:refnum<class "Channel.lvclass">)  [unwired: 7 in]
                n1974 = call "Write section_name.vi"("error in (no error)"=w4800, "section_name"="CCD_ACS1", "Channel in"=w4799) -> ("error out"=w4801:errorcluster, "Channel out"=w4796:refnum<class "Channel.lvclass">)  [unwired: 7 in]
                n1975 = call-dynamic "save config.vi"("error in (no error)"=w4801, "file config"="lastsaved.cfg", "Channel in"=w4796) -> ("error out"=w4772:errorcluster, "Channel out"=w4771:refnum<class "Channel.lvclass">)  [unwired: 7 in]
                n1976 = local read "Filter1"() -> (w4773:u8)
                n1977 = call-dynamic "Write Filter.vi"("error in (no error)"=w4772, "Filter"=w4773, "Channel in"=w4771) -> ("error out"=w4788:errorcluster, "Channel out"=w4787:refnum<class "Channel.lvclass">)  [unwired: 7 in]
                n1978 = call-dynamic "Read Interface.vi"("error in (no error)"=w4788, "Channel in"=w4787) -> ("error out"=w4784:errorcluster, "Interface.lvclass"=w4783:refnum<class "Interface.lvclass">, "Channel out"=w4777:refnum<class "Channel.lvclass">)  [unwired: 7 in]
                n1979 = call-dynamic "Write Suffix.vi"("error in (no error)"=w4784, "Suffix"=w4760, "Interface in"=w4783) -> ("error out"=w4774:errorcluster, "Interface out"=w4778:refnum<class "Interface.lvclass">)  [unwired: 7 in]
                n1980 = call-dynamic "Write ObsType.vi"("error in (no error)"=w4774, "ObsType"=w4759, "Interface in"=w4778) -> ("error out"=w4775:errorcluster, "Interface out"=w4779:refnum<class "Interface.lvclass">)  [unwired: 7 in]
                n1981 = call-dynamic "Write Object.vi"("error in (no error)"=w4775, "Object"=w4768, "Interface in"=w4779) -> ("error out"=w4776:errorcluster, "Interface out"=w4780:refnum<class "Interface.lvclass">)  [unwired: 7 in]
                n1982 = call-dynamic "Write Comments.vi"("error in (no error)"=w4776, "Comments"=w4767, "Interface in"=w4780) -> ("error out"=w4781:errorcluster, "Interface out"=w4782:refnum<class "Interface.lvclass">)  [unwired: 7 in]
                n1983 = call-dynamic "Write Observer.vi"("error in (no error)"=w4781, "Observer"=w4766, "Interface in"=w4782) -> ("error out"=w4786:errorcluster, "Interface out"=w4785:refnum<class "Interface.lvclass">)  [unwired: 7 in]
                n1984 = call-dynamic "Write Interface.vi"("error in (no error)"=w4786, "Interface.lvclass"=w4785, "Channel in"=w4777) -> ("error out"=w4769:errorcluster, "Channel out"=w4770:refnum<class "Channel.lvclass">)  [unwired: 7 in]
                n1985 = call-dynamic "Read State Machine.vi"("error in (no error)"=w4769, "Device in"=w4770) -> ("error out"=w4804:errorcluster, "State Machine.lvclass"=w4794:refnum<class "State Machine.lvclass">, "Device out"=w4795:refnum<class "Channel.lvclass">)  [unwired: 7 in]
                n1986 = call-dynamic "Write State.vi"("error in (no error)"=w4804, "State"=60, "State Machine in"=w4794) -> ("error out"=w4803:errorcluster, "State Machine out"=w4793:refnum<class "State Machine.lvclass">)  [unwired: 7 in]
                n1987 = call-dynamic "Write State Machine.vi"("error in (no error)"=w4803, "State Machine.lvclass"=w4793, "Device in"=w4795) -> ("error out"=w4791:errorcluster, "Device out"=w4792:refnum<class "Channel.lvclass">)  [unwired: 7 in]
                n1988 = call-dynamic "Write Channel.vi"("error in (no error)"=w4791, "Channel.lvclass"=w4792, "Acquisition in"=w4820) -> ("error out"=w4817:errorcluster, "Acquisition out"=w4816:refnum<class "Acquisition.lvclass">)  [unwired: 7 in]
              }
            }
            n1989 = case shown="True" w4497 {
              tunnel: w4499 -> [w4673 w4712]
              tunnel: w4498 -> [w4672 w4711]
              tunnel: [w4673 w4710] -> w4510
              tunnel: [w4672 w4709] -> w4509
              tunnel: w4484 -> [_ w4688]
              tunnel: w4483 -> [_ w4687]
              tunnel: w4482 -> [_ w4686]
              tunnel: w4481 -> [_ w4680]
              tunnel: w4480 -> [_ w4679]
              frame False {
              }
              frame True {
                # "nome do arquivo .cfg"
                # "seção no arquivo .cfg"
                # "open"
                n1990 = call-dynamic "Read Channel.vi"("error in (no error)"=w4711, "Acquisition in"=w4712) -> ("error out"=w4716:errorcluster, "Channel.lvclass"=w4715:refnum<class "Channel.lvclass">, "Acquisition out"=w4714:refnum<class "Acquisition.lvclass">)  [unwired: 7 in]
                n1991 = call-dynamic "Read Interface.vi"("error in (no error)"=w4716, "Channel in"=w4715) -> ("error out"=w4676:errorcluster, "Interface.lvclass"=w4678:refnum<class "Interface.lvclass">, "Channel out"=w4713:refnum<class "Channel.lvclass">)  [unwired: 7 in]
                n1992 = call-dynamic "Read restoreExpTime.vi"("error in (no error)"=w4676, "Interface in"=w4678) -> ("error out"=w4675:errorcluster, "restoreExpTime"=w4674:bool, "Interface out"=w4677:refnum<class "Interface.lvclass">)  [unwired: 7 in]
                n1993 = case shown="True" w4674 {
                  tunnel: w4677 -> [w4743 w4748]
                  tunnel: [w4743 w4751] -> w4682
                  tunnel: w4675 -> [w4742 w4747]
                  tunnel: [w4742 w4750] -> w4681
                  frame False {
                  }
                  frame True {
                    n1994 = call-dynamic "Write restoreExpTime.vi"("error in (no error)"=w4747, "restoreExpTime"=FALSE, "Interface in"=w4748) -> ("error out"=w4745:errorcluster, "Interface out"=w4746:refnum<class "Interface.lvclass">)  [unwired: 7 in]
                    n1995 = call-dynamic "Read prev ExpTime.vi"("error in (no error)"=w4745, "Interface in"=w4746) -> ("error out"=w4750:errorcluster, "prev ExpTime"=w4749:dbl, "Interface out"=w4751:refnum<class "Interface.lvclass">)  [unwired: 7 in]
                    n1996 = property on="Exptime ch2" class="DigNum (strict)"("Value"=w4749) -> ()  [unwired: 2 in, 2 out]
                  }
                }
                n1997 = call-dynamic "Read PREV_FT.vi"("error in (no error)"=w4681, "Interface in"=w4682) -> ("error out"=w4684:errorcluster, "PREV_FT"=w4683:bool, "Interface out"=w4685:refnum<class "Interface.lvclass">)  [unwired: 7 in]
                n1998 = call-dynamic "Get CCD_Config.vi"("error in (no error)"=w4684, "Interface in"=w4685) -> ("error out"=w4721:errorcluster, "output cluster"=w4720:T24, "Interface out"=w4724:refnum<class "Interface.lvclass">)  [unwired: 7 in]
                n1999 = Bundle By Name(cluster=w4720, "SHUTTER_MODE"=u8 1, "FRAME_TRANSFER"=w4683) -> (w4722:T24)
                n2000 = call-dynamic "Set CCD_Config.vi"("error in (no error)"=w4721, "input cluster"=w4722, "Interface in"=w4724) -> ("error out"=w4719:errorcluster, "Interface out"=w4725:refnum<class "Interface.lvclass">)  [unwired: 7 in]
                n2001 = Flatten To String(anything=w4722, error in (no error)=w4719) -> (data string=w4717:string, error out=w4718:errorcluster)  [unwired: 2 in, 1 out]
                n2002 = call "Write flatted cluster.vi"("error in (no error)"=w4718, "flatted cluster"=w4717, "Interface in"=w4725) -> ("error out"=w4727:errorcluster, "Interface out"=w4726:refnum<class "Interface.lvclass">)  [unwired: 7 in]
                n2003 = call-dynamic "Write Interface.vi"("error in (no error)"=w4727, "Interface.lvclass"=w4726, "Channel in"=w4713) -> ("error out"=w4732:errorcluster, "Channel out"=w4733:refnum<class "Channel.lvclass">)  [unwired: 7 in]
                n2004 = call "Write section_name.vi"("error in (no error)"=w4732, "section_name"="CCD_ACS2", "Channel in"=w4733) -> ("error out"=w4731:errorcluster, "Channel out"=w4736:refnum<class "Channel.lvclass">)  [unwired: 7 in]
                n2005 = call-dynamic "save config.vi"("error in (no error)"=w4731, "file config"="lastsaved.cfg", "Channel in"=w4736) -> ("error out"=w4690:errorcluster, "Channel out"=w4695:refnum<class "Channel.lvclass">)  [unwired: 7 in]
                n2006 = local read "Filter2"() -> (w4689:u8)
                n2007 = call-dynamic "Write Filter.vi"("error in (no error)"=w4690, "Filter"=w4689, "Channel in"=w4695) -> ("error out"=w4708:errorcluster, "Channel out"=w4694:refnum<class "Channel.lvclass">)  [unwired: 7 in]
                n2008 = call-dynamic "Read Interface.vi"("error in (no error)"=w4708, "Channel in"=w4694) -> ("error out"=w4705:errorcluster, "Interface.lvclass"=w4704:refnum<class "Interface.lvclass">, "Channel out"=w4693:refnum<class "Channel.lvclass">)  [unwired: 7 in]
                n2009 = call-dynamic "Write Suffix.vi"("error in (no error)"=w4705, "Suffix"=w4680, "Interface in"=w4704) -> ("error out"=w4696:errorcluster, "Interface out"=w4699:refnum<class "Interface.lvclass">)  [unwired: 7 in]
                n2010 = call-dynamic "Write ObsType.vi"("error in (no error)"=w4696, "ObsType"=w4679, "Interface in"=w4699) -> ("error out"=w4697:errorcluster, "Interface out"=w4700:refnum<class "Interface.lvclass">)  [unwired: 7 in]
                n2011 = call-dynamic "Write Object.vi"("error in (no error)"=w4697, "Object"=w4688, "Interface in"=w4700) -> ("error out"=w4698:errorcluster, "Interface out"=w4701:refnum<class "Interface.lvclass">)  [unwired: 7 in]
                n2012 = call-dynamic "Write Comments.vi"("error in (no error)"=w4698, "Comments"=w4687, "Interface in"=w4701) -> ("error out"=w4702:errorcluster, "Interface out"=w4703:refnum<class "Interface.lvclass">)  [unwired: 7 in]
                n2013 = call-dynamic "Write Observer.vi"("error in (no error)"=w4702, "Observer"=w4686, "Interface in"=w4703) -> ("error out"=w4707:errorcluster, "Interface out"=w4706:refnum<class "Interface.lvclass">)  [unwired: 7 in]
                n2014 = call-dynamic "Write Interface.vi"("error in (no error)"=w4707, "Interface.lvclass"=w4706, "Channel in"=w4693) -> ("error out"=w4691:errorcluster, "Channel out"=w4692:refnum<class "Channel.lvclass">)  [unwired: 7 in]
                n2015 = call-dynamic "Read State Machine.vi"("error in (no error)"=w4691, "Device in"=w4692) -> ("error out"=w4728:errorcluster, "State Machine.lvclass"=w4738:refnum<class "State Machine.lvclass">, "Device out"=w4737:refnum<class "Channel.lvclass">)  [unwired: 7 in]
                n2016 = call-dynamic "Write State.vi"("error in (no error)"=w4728, "State"=60, "State Machine in"=w4738) -> ("error out"=w4729:errorcluster, "State Machine out"=w4739:refnum<class "State Machine.lvclass">)  [unwired: 7 in]
                n2017 = call-dynamic "Write State Machine.vi"("error in (no error)"=w4729, "State Machine.lvclass"=w4739, "Device in"=w4737) -> ("error out"=w4741:errorcluster, "Device out"=w4740:refnum<class "Channel.lvclass">)  [unwired: 7 in]
                n2018 = call-dynamic "Write Channel.vi"("error in (no error)"=w4741, "Channel.lvclass"=w4740, "Acquisition in"=w4714) -> ("error out"=w4709:errorcluster, "Acquisition out"=w4710:refnum<class "Acquisition.lvclass">)  [unwired: 7 in]
              }
            }
            n2019 = case shown="True" w4494 {
              tunnel: w4496 -> [w4593 w4632]
              tunnel: w4495 -> [w4592 w4631]
              tunnel: [w4593 w4630] -> w4508
              tunnel: [w4592 w4629] -> w4507
              tunnel: w4484 -> [_ w4608]
              tunnel: w4483 -> [_ w4607]
              tunnel: w4482 -> [_ w4606]
              tunnel: w4481 -> [_ w4600]
              tunnel: w4480 -> [_ w4599]
              frame False {
              }
              frame True {
                # "nome do arquivo .cfg"
                # "seção no arquivo .cfg"
                # "open"
                n2020 = call-dynamic "Read Channel.vi"("error in (no error)"=w4631, "Acquisition in"=w4632) -> ("error out"=w4636:errorcluster, "Channel.lvclass"=w4635:refnum<class "Channel.lvclass">, "Acquisition out"=w4634:refnum<class "Acquisition.lvclass">)  [unwired: 7 in]
                n2021 = call-dynamic "Read Interface.vi"("error in (no error)"=w4636, "Channel in"=w4635) -> ("error out"=w4596:errorcluster, "Interface.lvclass"=w4598:refnum<class "Interface.lvclass">, "Channel out"=w4633:refnum<class "Channel.lvclass">)  [unwired: 7 in]
                n2022 = call-dynamic "Read restoreExpTime.vi"("error in (no error)"=w4596, "Interface in"=w4598) -> ("error out"=w4595:errorcluster, "restoreExpTime"=w4594:bool, "Interface out"=w4597:refnum<class "Interface.lvclass">)  [unwired: 7 in]
                n2023 = case shown="True" w4594 {
                  tunnel: w4597 -> [w4663 w4668]
                  tunnel: [w4663 w4671] -> w4602
                  tunnel: w4595 -> [w4662 w4667]
                  tunnel: [w4662 w4670] -> w4601
                  frame False {
                  }
                  frame True {
                    n2024 = call-dynamic "Write restoreExpTime.vi"("error in (no error)"=w4667, "restoreExpTime"=FALSE, "Interface in"=w4668) -> ("error out"=w4665:errorcluster, "Interface out"=w4666:refnum<class "Interface.lvclass">)  [unwired: 7 in]
                    n2025 = call-dynamic "Read prev ExpTime.vi"("error in (no error)"=w4665, "Interface in"=w4666) -> ("error out"=w4670:errorcluster, "prev ExpTime"=w4669:dbl, "Interface out"=w4671:refnum<class "Interface.lvclass">)  [unwired: 7 in]
